vi "H(w) from IIR Cluster.vi"(10 "w":dbl format="%.2f", 11 "IIR Filter Cluster":T1 {"Forward Coefficients" format="%.4f"; "Reverse Coefficients" format="%.4f"}) -> (3 "Complex response":cdb)   [LabVIEW 2014, in "NI_AALBase.lvlib"]
uses:
  NI_AALBase.lvlib
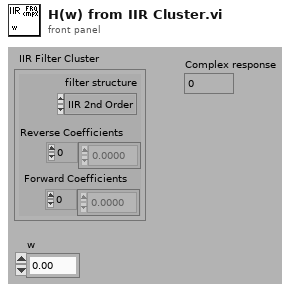
[diagram p1: front panel]
types:
  T1 = cluster{"filter structure":enum32{"IIR 2nd Order", "IIR 4th Order"}, "Reverse Coefficients":dbl[], "Forward Coefficients":dbl[]}
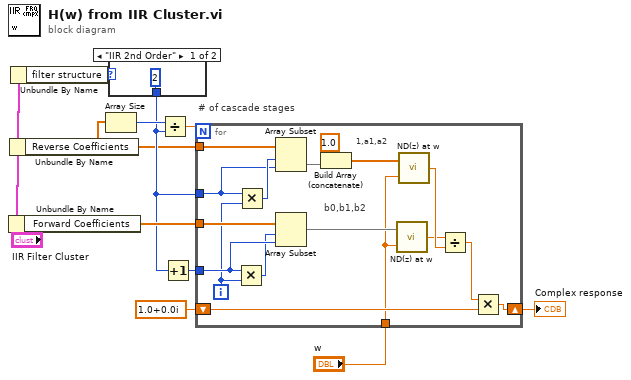
[diagram p0: block diagram]
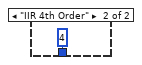
[diagram p2: hidden frame]
diagram:
  # "# of cascade stages"
  n1 = Unbundle By Name("IIR Filter Cluster") -> ("Forward Coefficients"=w9:dbl[])
  n2 = Unbundle By Name("IIR Filter Cluster") -> ("Reverse Coefficients"=w5:dbl[])
  n3 = Unbundle By Name("IIR Filter Cluster") -> ("filter structure"=w11:enum32{"IIR 2nd Order", "IIR 4th Order"})
  n4 = Array Size(array=w5) -> (size(s)=w10:i32)
  n5 = case shown="\"IIR 2nd Order\"" w11 {
    tunnel: [2 4] -> w7
    frame "IIR 2nd Order" {
    }
    frame "IIR 4th Order" {
    }
  }
  n6 = Divide(x=w10, y=w7) -> (x/y=w6:dbl)
  n7 = Increment(x=w7) -> (x+1=w4:i32)
  n8 = for {
    N: w6 -> [_]
    shift-right: [w21] -> w1
    shift-left: cdb 1.0+0.0i -> [w19]
    tunnel: w7 -> [w27]
    tunnel: w5 -> [w26]
    tunnel: w9 -> [w25]
    tunnel: w4 -> [w24]
    tunnel: "w" -> [w16]
    i -> [w22]
    # "b0,b1,b2"
    # "1,a1,a2"
    n9 = Multiply(x=w24, y=w22) -> (x*y=w23:i32)
    n10 = Multiply(x=w27, y=w22) -> (x*y=w28:i32)
    n11 = Array Subset(array=w26, index=w28, length=w27) -> (w30:dbl[])
    n12 = Array Subset(array=w25, index=w23, length=w24) -> (w17:dbl[])
    n13 = Build Array (concatenate)(1.0, w30) -> (w18:dbl[])
    n14 = call "ND(z) at w.vi"("w"=w16, "ND(z)"=w17) -> ("ND(w)"=w14:cdb)
    n15 = call "ND(z) at w.vi"("w"=w16, "ND(z)"=w18) -> ("ND(w)"=w15:cdb)
    n16 = Divide(x=w14, y=w15) -> (x/y=w20:cdb)
    n17 = Multiply(x=w20, y=w19) -> (x*y=w21:cdb)
  }
  "Complex response" <- w1
